vi "A01423754_Ximena_Avila_Ejercicio_04_conversion_de_bases_17_Enero.vi"() -> ()   [LabVIEW 2018]
panel:
  in  "Numero":string
  out "Nuevo numero":string
  in  "Nueva base":u64
  in  "Base":u64
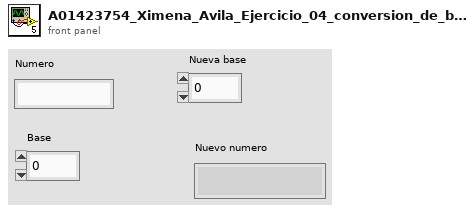
[diagram p1: front panel]
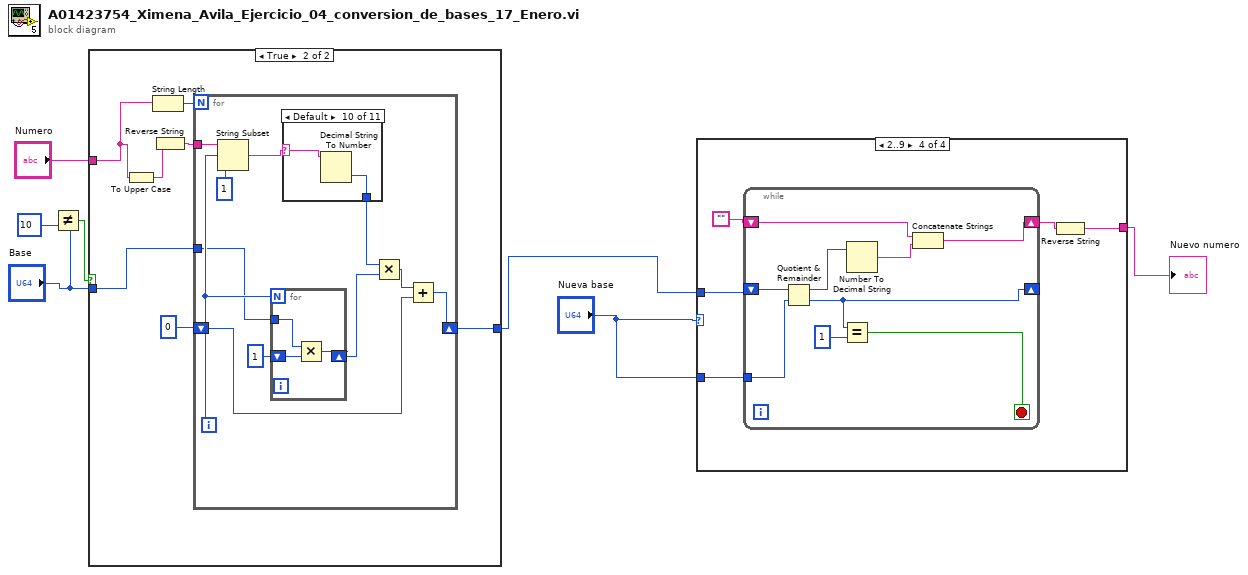
[diagram p0: block diagram]
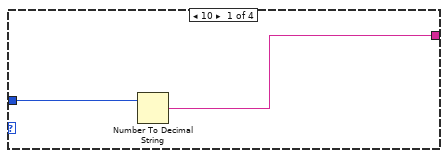
[diagram p2: hidden frame]
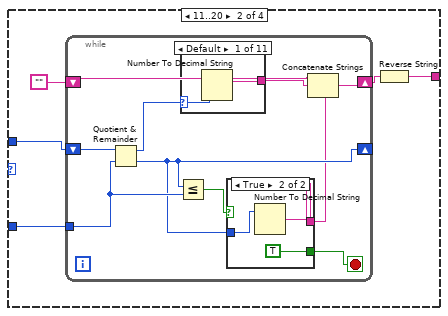
[diagram p3: hidden frame]
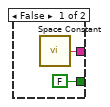
[diagram p4: hidden frame]
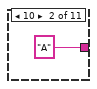
[diagram p5: hidden frame]
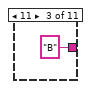
[diagram p6: hidden frame]
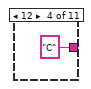
[diagram p7: hidden frame]
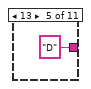
[diagram p8: hidden frame]
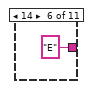
[diagram p9: hidden frame]
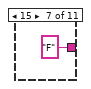
[diagram p10: hidden frame]
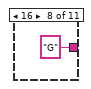
[diagram p11: hidden frame]
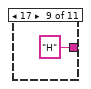
[diagram p12: hidden frame]
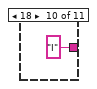
[diagram p13: hidden frame]
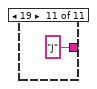
[diagram p14: hidden frame]
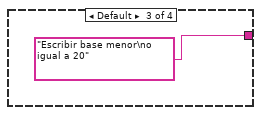
[diagram p15: hidden frame]
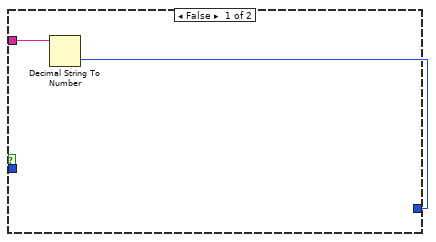
[diagram p16: hidden frame]
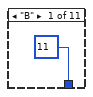
[diagram p17: hidden frame]
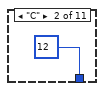
[diagram p18: hidden frame]
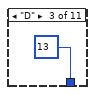
[diagram p19: hidden frame]
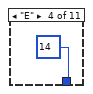
[diagram p20: hidden frame]
diagram:
  n1 = Not Equal?(x="Base", y=u64 10) -> (x != y?=w6:bool)
  n2 = case shown="True" w6 {
    tunnel: "Base" -> [_ w15]
    tunnel: [w8 w14] -> w3
    tunnel: "Numero" -> [w9 w10]
    frame False {
      n3 = Decimal String To Number(string=w9) -> (number=w8:i32)  [unwired: 2 in, 1 out]
    }
    frame True {
      n4 = To Upper Case(1:w10) -> (0:w11:string)
      n5 = String Length(string=w10) -> (length=w16:i32)
      n6 = Reverse String(1:w11) -> (0:w13:string)
      n7 = for {
        N: w16 -> [_]
        tunnel: w15 -> [w25]
        shift-right: [w22] -> w14
        shift-left: 0 -> [w21]
        tunnel: w13 -> [w19]
        i -> [w26]
        n8 = String Subset(string=w19, offset (0)=w26, length (rest)=1 ("length (rest)")) -> (substring=w18:string)
        n9 = for {
          N: w26 -> [_]
          tunnel: w25 -> [w42]
          shift-right: [w41] -> w24
          shift-left: u64 1 -> [w40]
          n10 = Multiply(x=w42, y=w40) -> (x*y=w41:u64)
        }
        n11 = case shown="Default" w18 {
          selector: w18 -> [_ _ _ _ _ _ _ _ _ w37 _]
          tunnel: [11 12 13 14 15 16 17 18 19 w38 10] -> w17
          frame "B" {
          }
          frame "C" {
          }
          frame "D" {
          }
          frame "E" {
          }
          frame "F" {
          }
          frame "G" {
          }
          frame "H" {
          }
          frame "I" {
          }
          frame "J" {
          }
          frame Default {
            n12 = Decimal String To Number(string=w37) -> (number=w38:i32)  [unwired: 2 in, 1 out]
          }
          frame "A" {
          }
        }
        n13 = Multiply(x=w17, y=w24) -> (x*y=w23:u64)
        n14 = Add(x=w23, y=w21) -> (x+y=w22:u64)
      }
    }
  }
  n15 = case shown="2..9" "Nueva base" {
    tunnel: w3 -> [w44 w49 _ w82]
    tunnel: [w43 w46 "Escribir base menor\no igual a 20" w79] -> w4
    tunnel: "Nueva base" -> [_ w48 _ w81]
    frame 10 {
      n16 = Number To Decimal String(number=w44) -> (decimal integer string=w43:string)  [unwired: 1 in]
    }
    frame 11..20 {
      n17 = while {
        shift-right: [w52] -> _
        shift-left: w49 -> [w59]
        tunnel: w48 -> [w54]
        shift-right: [w57] -> w47
        shift-left: "" -> [w56]
        stop <- w50 stop-if-true
        n18 = Quotient & Remainder(x=w59, y=w54) -> (x-y*floor(x/y)=w55:u64, floor(x/y)=w52:u64)
        n19 = Less Or Equal?(x=w52, y=w54) -> (x <= y?=w53:bool)
        n20 = case shown="Default" w55 {
          selector: w55 -> [w66 _ _ _ _ _ _ _ _ _ _]
          tunnel: [w65 "A" "B" "C" "D" "E" "F" "G" "H" "I" "J"] -> w58
          frame Default {
            n21 = Number To Decimal String(number=w66) -> (decimal integer string=w65:string)  [unwired: 1 in]
          }
          frame 10 {
          }
          frame 11 {
          }
          frame 12 {
          }
          frame 13 {
          }
          frame 14 {
          }
          frame 15 {
          }
          frame 16 {
          }
          frame 17 {
          }
          frame 18 {
          }
          frame 19 {
          }
        }
        n22 = case shown="True" w53 {
          tunnel: w52 -> [_ w64]
          tunnel: [w60 w63] -> w51
          tunnel: [FALSE TRUE] -> w50
          frame False {
            n23 = call <vilib>:"Space Constant.vi"() -> ("String"=w60:string)
          }
          frame True {
            n24 = Number To Decimal String(number=w64) -> (decimal integer string=w63:string)  [unwired: 1 in]
          }
        }
        n25 = Concatenate Strings(w56, w58, w51) -> (w57:string)
      }
      n26 = Reverse String(1:w47) -> (0:w46:string)
    }
    frame Default {
    }
    frame 2..9 {
      n27 = while {
        shift-right: [w87] -> _
        shift-left: w82 -> [w91]
        tunnel: w81 -> [w90]
        shift-right: [w84] -> w78
        shift-left: "" -> [w85]
        stop <- w83 stop-if-true
        n28 = Quotient & Remainder(x=w91, y=w90) -> (x-y*floor(x/y)=w88:u64, floor(x/y)=w87:u64)
        n29 = Equal?(x=w87, y=u64 1) -> (x = y?=w83:bool)
        n30 = Number To Decimal String(number=w88) -> (decimal integer string=w86:string)  [unwired: 1 in]
        n31 = Concatenate Strings(w85, w86) -> (w84:string)
      }
      n32 = Reverse String(1:w78) -> (0:w79:string)
    }
  }
  "Nuevo numero" <- w4
